vi "GetPortNo.vi"(9 "External":i32(ring) items=["GENERAL OUT", "GENERAL IN", "SYNC OUT", "SYNC IN "], 10 "Device Code":u32) -> (1 "Port No.":i32)   [LabVIEW 8.6]
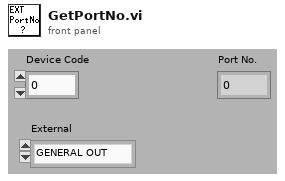
[diagram p1: front panel]
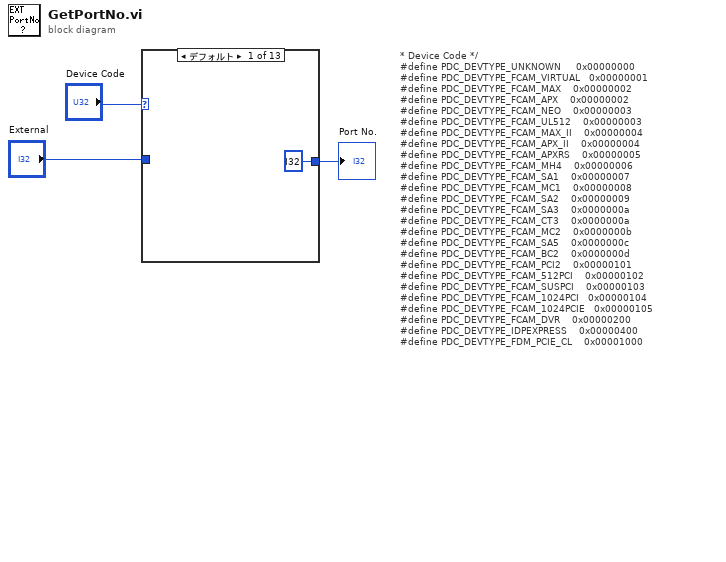
[diagram p0: block diagram]
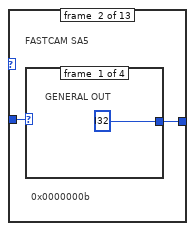
[diagram p2: hidden frame]
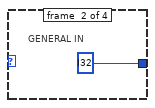
[diagram p3: hidden frame]
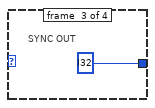
[diagram p4: hidden frame]
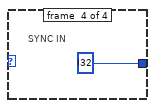
[diagram p5: hidden frame]
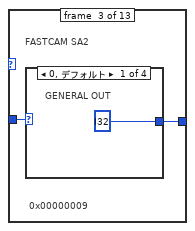
[diagram p6: hidden frame]
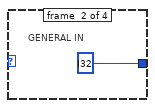
[diagram p7: hidden frame]
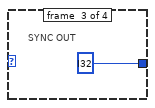
[diagram p8: hidden frame]
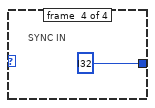
[diagram p9: hidden frame]
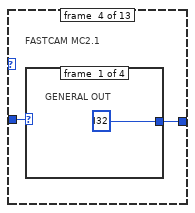
[diagram p10: hidden frame]
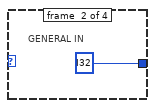
[diagram p11: hidden frame]
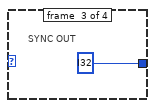
[diagram p12: hidden frame]
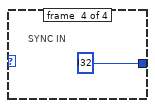
[diagram p13: hidden frame]
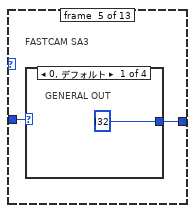
[diagram p14: hidden frame]
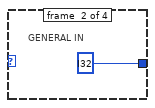
[diagram p15: hidden frame]
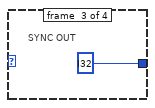
[diagram p16: hidden frame]
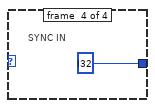
[diagram p17: hidden frame]
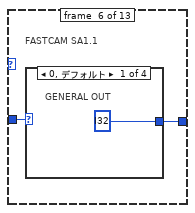
[diagram p18: hidden frame]
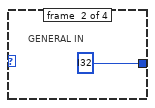
[diagram p19: hidden frame]
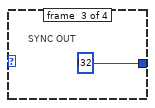
[diagram p20: hidden frame]
diagram:
  # "*\tDevice Code\t*/\n#define\tPDC_DEVTYPE_UNKNOWN\t\t\t\t\t0x00000000\n#define\tPDC_DEVTYPE_FCAM_VIRTUAL\t\t\t0x00000001\n#define\tPDC_DEVTYPE_FCAM_MAX\t\t\t\t0x00000002\n#define\tPDC_DEVTYPE_FCAM_APX\t\t\t\t0x00000002\n#define\tPDC_DEVTYPE_FCAM_NEO\t\t\t\t0x00000003\n#define\tPDC_DEVTYPE_FCAM_UL512\t\t\t\t0x00000003\n#define\tPDC_DEVTYPE_FCAM_MAX_II\t\t\t\t0x00000004\n#define\tPDC_DEVTYPE_FCAM_APX_II\t\t\t\t0x00000004\n#define\tPDC_DEVTYPE_FCAM_APXRS\t\t\t\t0x00000005\n#define\tPDC_DEVTYPE_FCAM_MH4\t\t\t\t0x00000006\n#define\tPDC_DEVTYPE_FCAM_SA1\t\t\t\t0x00000007\n#define\tPDC_DEVTYPE_FCAM_MC1\t\t\t\t0x00000008\n#define\tPDC_DEVTYPE_FCAM_SA2\t\t\t\t0x00000009\n#define\tPDC_DEVTYPE_FCAM_SA3\t\t\t\t0x0000000a\n#define\tPDC_DEVTYPE_FCAM_CT3\t\t\t\t0x0000000a\n#define\tPDC_DEVTYPE_FCAM_MC2\t\t\t\t0x0000000b\n#define\tPDC_DEVTYPE_FCAM_SA5\t\t\t\t0x0000000c\n#define\tPDC_DEVTYPE_FCAM_BC2\t\t\t\t0x0000000d\n#define\tPDC_DEVTYPE_FCAM_PCI2\t\t\t\t0x00000101\n#define\tPDC_DEVTYPE_FCAM_512PCI\t\t\t\t0x00000102\n#define\tPDC_DEVTYPE_FCAM_SUSPCI\t\t\t\t0x00000103\n#define\tPDC_DEVTYPE_FCAM_1024PCI\t\t\t0x00000104\n#define\tPDC_DEVTYPE_FCAM_1024PCIE\t\t\t0x00000105\n#define PDC_DEVTYPE_FCAM_DVR\t\t\t\t0x00000200\n#define\tPDC_DEVTYPE_IDPEXPRESS\t\t\t\t0x00000400\n#define\tPDC_DEVTYPE_FDM_PCIE_CL\t\t\t\t0x00001000"
  n1 = case shown="デフォルト" "Device Code" {
    tunnel: "External" -> [_ w6 w12 w18 w24 w30 w36 w42 w48 w54 w60 w66 w72]
    tunnel: [i32 ? ("Port No.") w5 w11 w17 w23 w29 w35 w41 w47 w53 w59 w65 w71] -> w1
    frame #0 {
    }
    frame #1 {
      # "0x0000000b"
      # "FASTCAM SA5"
      n2 = case shown="3" w6 {
        tunnel: [i32 ? ("Port No.") i32 ? ("Port No.") i32 ? ("Port No.") i32 ? ("Port No.")] -> w5
        frame #0 {
          # "GENERAL OUT"
        }
        frame #1 {
          # "GENERAL IN"
        }
        frame #2 {
          # "SYNC OUT"
        }
        frame #3 {
          # "SYNC IN"
        }
      }
    }
    frame #2 {
      # "0x00000009"
      # "FASTCAM SA2"
      n3 = case shown="0, デフォルト" w12 {
        tunnel: [i32 ? ("Port No.") i32 ? ("Port No.") i32 ? ("Port No.") i32 ? ("Port No.")] -> w11
        frame #0 {
          # "GENERAL OUT"
        }
        frame #1 {
          # "GENERAL IN"
        }
        frame #2 {
          # "SYNC OUT"
        }
        frame #3 {
          # "SYNC IN"
        }
      }
    }
    frame #3 {
      # "FASTCAM MC2.1"
      n4 = case shown="3" w18 {
        tunnel: [i32 ? ("Port No.") i32 ? ("Port No.") i32 ? ("Port No.") i32 ? ("Port No.")] -> w17
        frame #0 {
          # "GENERAL OUT"
        }
        frame #1 {
          # "GENERAL IN"
        }
        frame #2 {
          # "SYNC OUT"
        }
        frame #3 {
          # "SYNC IN"
        }
      }
    }
    frame #4 {
      # "FASTCAM SA3"
      n5 = case shown="0, デフォルト" w24 {
        tunnel: [i32 ? ("Port No.") i32 ? ("Port No.") i32 ? ("Port No.") i32 ? ("Port No.")] -> w23
        frame #0 {
          # "GENERAL OUT"
        }
        frame #1 {
          # "GENERAL IN"
        }
        frame #2 {
          # "SYNC OUT"
        }
        frame #3 {
          # "SYNC IN"
        }
      }
    }
    frame #5 {
      # "FASTCAM SA1.1"
      n6 = case shown="0, デフォルト" w30 {
        tunnel: [i32 ? ("Port No.") i32 ? ("Port No.") i32 ? ("Port No.") i32 ? ("Port No.")] -> w29
        frame #0 {
          # "GENERAL OUT"
        }
        frame #1 {
          # "GENERAL IN"
        }
        frame #2 {
          # "SYNC OUT"
        }
        frame #3 {
          # "SYNC IN"
        }
      }
    }
    frame #6 {
      # "FASTCAM MH4"
      n7 = case shown="0, デフォルト" w36 {
        tunnel: [i32 ? ("Port No.") i32 ? ("Port No.") i32 ? ("Port No.") i32 ? ("Port No.")] -> w35
        frame #0 {
          # "GENERAL OUT"
        }
        frame #1 {
          # "GENERAL IN"
        }
        frame #2 {
          # "SYNC OUT"
        }
        frame #3 {
          # "SYNC IN"
        }
      }
    }
    frame #7 {
      # "FASTCAM APX RS"
      n8 = case shown="0, デフォルト" w42 {
        tunnel: [i32 ? ("Port No.") i32 ? ("Port No.") i32 ? ("Port No.") i32 ? ("Port No.")] -> w41
        frame #0 {
          # "GENERAL OUT"
        }
        frame #1 {
          # "GENERAL IN"
        }
        frame #2 {
          # "SYNC OUT"
        }
        frame #3 {
          # "SYNC IN"
        }
      }
    }
    frame #8 {
      # "FASTCAM MAX"
      n9 = case shown="0, デフォルト" w48 {
        tunnel: [i32 ? ("Port No.") i32 ? ("Port No.") i32 ? ("Port No.") i32 ? ("Port No.")] -> w47
        frame #0 {
          # "GENERAL OUT"
        }
        frame #1 {
          # "GENERAL IN"
        }
        frame #2 {
          # "SYNC OUT"
        }
        frame #3 {
          # "SYNC IN"
        }
      }
    }
    frame #9 {
      # "FASTCAM NEO"
      n10 = case shown="0, デフォルト" w54 {
        tunnel: [i32 ? ("Port No.") i32 ? ("Port No.") i32 ? ("Port No.") i32 ? ("Port No.")] -> w53
        frame #0 {
          # "GENERAL OUT"
        }
        frame #1 {
          # "GENERAL IN"
        }
        frame #2 {
          # "SYNC OUT"
        }
        frame #3 {
          # "SYNC IN"
        }
      }
    }
    frame #10 {
      # "FASTCAM MC1"
      n11 = case shown="3" w60 {
        tunnel: [i32 ? ("Port No.") i32 ? ("Port No.") i32 ? ("Port No.") i32 ? ("Port No.")] -> w59
        frame #0 {
          # "GENERAL OUT"
        }
        frame #1 {
          # "GENERAL IN"
        }
        frame #2 {
          # "SYNC OUT"
        }
        frame #3 {
          # "SYNC IN"
        }
      }
    }
    frame #11 {
      # "FASTCAM 1024PCI"
      n12 = case shown="3" w66 {
        tunnel: [i32 ? ("Port No.") i32 ? ("Port No.") i32 ? ("Port No.") i32 ? ("Port No.")] -> w65
        frame #0 {
          # "GENERAL OUT"
        }
        frame #1 {
          # "GENERAL IN"
        }
        frame #2 {
          # "SYNC OUT"
        }
        frame #3 {
          # "SYNC IN"
        }
      }
    }
    frame #12 {
      # "FASTCAM 512PCI"
      n13 = case shown="3" w72 {
        tunnel: [i32 ? ("Port No.") i32 ? ("Port No.") i32 ? ("Port No.") i32 ? ("Port No.")] -> w71
        frame #0 {
          # "GENERAL OUT"
        }
        frame #1 {
          # "GENERAL IN"
        }
        frame #2 {
          # "SYNC OUT"
        }
        frame #3 {
          # "SYNC IN"
        }
      }
    }
  }
  "Port No." <- w1
